vi "Initialize DAQ1.vi"(10 "rate":dbl=1000.0, 11 "number of samples":i32=100) -> (0 "error out":errorcluster, 2 "cDAQ Dev SN":u32, 3 "task out":refnum<k21>)   [LabVIEW 2019]
uses:
  <vilib>/DAQmx/create/channels.llb/DAQmx Create Channel (AI-Voltage-Basic).vi
  <vilib>/DAQmx/create/channels.llb/DAQmx Create Channel (AI-Temperature-Thermocouple).vi
  <vilib>/DAQmx/configure/timing.llb/DAQmx Timing (Sample Clock).vi
  <resource>/objmgr/daqmx.rc
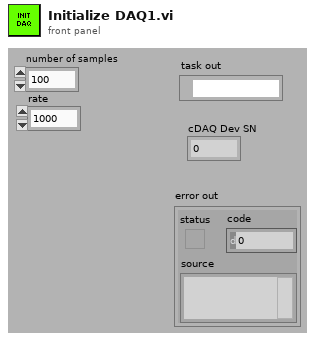
[diagram p1: front panel]
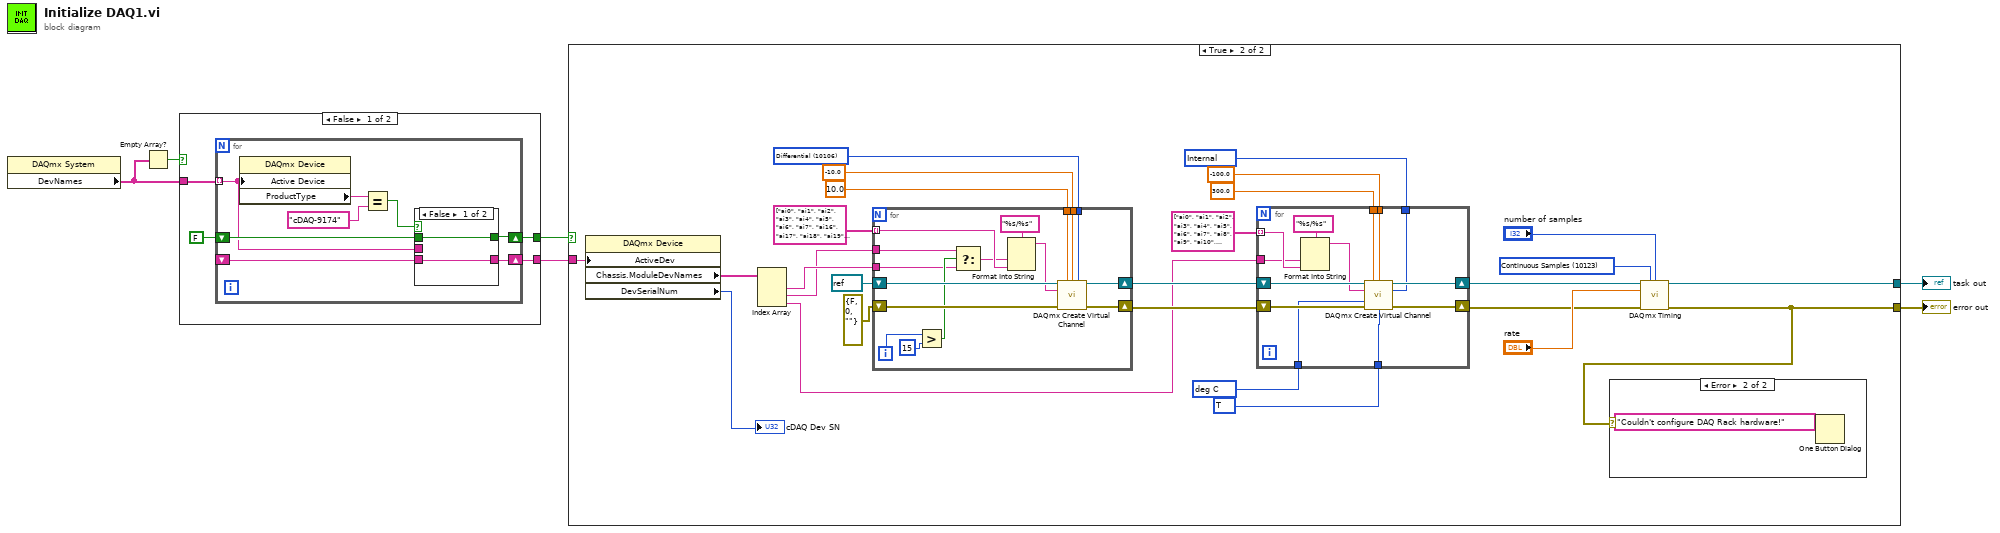
[diagram p0: block diagram]
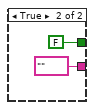
[diagram p3: hidden frame]
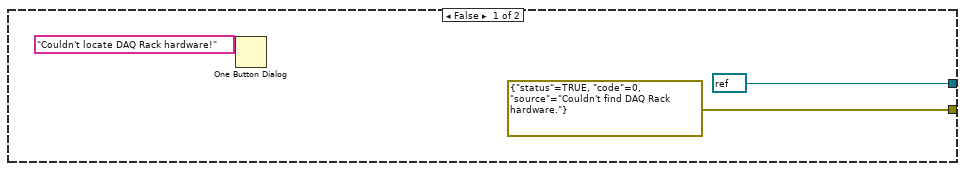
[diagram p4: hidden frame]
diagram:
  n1 = property class="DAQmx System"() -> ("DevNames"=w5:tag[])  [unwired: 2 in, 2 out]
  n2 = Empty Array?(array=w5) -> (empty?=w6:bool)
  n3 = case shown="False" w6 {
    tunnel: w5 -> [w10 _]
    tunnel: [w9 FALSE] -> w4
    tunnel: [w7 tag ""] -> w3
    frame False {
      n4 = for {
        tunnel: w10 -> [w14] mode=indexing
        shift-right: [w16] -> w9
        shift-left: FALSE -> [w15]
        shift-right: [w13] -> w7
        shift-left: _ -> [w12]
        n5 = property class="DAQmx Device"("Active Device"=w14) -> ("ProductType"=w11:string)  [unwired: 2 in, 2 out]
        n6 = Equal?(x=w11, y="cDAQ-9174" ("ProductType")) -> (x = y?=w17:bool)
        n7 = case shown="False" w17 {
          selector: w17 -> [_ w22]
          tunnel: [w20 w22] -> w16
          tunnel: w15 -> [w20 _]
          tunnel: [w19 w21] -> w13
          tunnel: w14 -> [_ w21]
          tunnel: w12 -> [w19 _]
          frame False {
          }
          frame True {
          }
        }
      }
    }
    frame True {
    }
  }
  n8 = case shown="True" w4 {
    tunnel: w3 -> [_ w35]
    tunnel: [refnum<k21> refnum ("task out") w36] -> w2
    tunnel: [errorcluster {"status"=TRUE, "code"=0, "source"="Couldn't find DAQ Rack hardware."} ("error out") w28] -> w1
    frame False {
      n9 = One Button Dialog(message="Couldn't locate DAQ Rack hardware!") -> ()  [unwired: 1 in, 1 out]
    }
    frame True {
      w40 = 10086 items=["J"=10072, "K"=10073, "N"=10077, "R"=10082, "S"=10085, "T"=10086, "B"=10047, "E"=10055] ("thermocouple type")
      w41 = 10143 items=["deg C"=10143, "deg F"=10144, "Kelvins"=10325, "deg R"=10145, "From Custom Scale"=10065] ("units")
      w44 = u32 10200 items=["Internal"=10200, "Constant Value"=10116, "Channel"=10113] ("cjc source")
      w47 = 10106 items=["default"=-1, "RSE"=10083, "NRSE"=10078, "Differential"=10106, "Pseudodifferential"=12529] ("input terminal configuration")
      w50 = 10123 items=["Finite Samples"=10178, "Continuous Samples"=10123, "Hardware Timed Single Point"=12522] ("sample mode")
      n10 = property class="DAQmx Device"("ActiveDev"=w35) -> ("Chassis.ModuleDevNames"=w34:tag[], "DevSerialNum"=→"cDAQ Dev SN":u32)  [unwired: 2 in, 2 out]
      n11 = Index Array(array=w34) -> (element #1=w32:tag, element #2=w31:tag, element #3=w33:tag)  [unwired: 3 in]
      n12 = for {
        tunnel: w47 -> [w82]
        tunnel: -10.0 ("minimum value") -> [w83]
        tunnel: 10.0 ("maximum value") -> [w84]
        tunnel: string[] ["ai0", "ai1", "ai2", "ai3", "ai4", "ai5", "ai6", "ai7", "ai16", "ai17", "ai18", "ai19", "ai20", "ai21", "ai22", "ai23", "ai0", "ai1", "ai2", "ai3", "ai4", "ai5", "ai6", "ai7", "ai16", "ai17", "ai18", "ai19", "ai20", "ai21", "ai22", "ai23"] ("Array") -> [w78] mode=indexing
        shift-right: [w69] -> w54
        shift-left: errorcluster {"status"=FALSE, "code"=0, "source"=""} ("error out") -> [w80]
        shift-right: [w79] -> w53
        shift-left: refnum<k21> refnum ("task out") -> [w81]
        tunnel: w32 -> [w72]
        tunnel: w31 -> [w71]
        i -> [w75]
        n13 = Greater?(x=w75, y=15) -> (0:w73:bool)
        n14 = Select(t=w71, s=w73, f=w72) -> (s? t:f=w70:tag)
        n15 = Format Into String(format string="%s/%s", w70, w78) -> (resulting string=w76:string)  [unwired: 2 in, 1 out]
        n16 = call-poly <vilib>:"DAQmx Create Virtual Channel.vi"("task in"=w81, "maximum value"=w84, "minimum value"=w83, "input terminal configuration"=w82, "physical channels"=w76, "error in"=w80) -> ("task out"=w79:refnum<k21>, "error out"=w69:errorcluster)  [unwired: 8 in]
      }
      n17 = for {
        tunnel: -100.0 ("minimum value") -> [w67]
        tunnel: 300.0 ("maximum value") -> [w68]
        tunnel: w40 -> [w60]
        tunnel: w41 -> [w62]
        tunnel: string[] ["ai0", "ai1", "ai2", "ai3", "ai4", "ai5", "ai6", "ai7", "ai8", "ai9", "ai10", "ai11", "ai12", "ai13", "ai14", "ai15"] ("Array") -> [w58] mode=indexing
        tunnel: w44 -> [w61]
        shift-right: [w63] -> w45
        shift-left: w54 -> [w65]
        shift-right: [w64] -> w46
        shift-left: w53 -> [w66]
        tunnel: w33 -> [w57]
        n18 = Format Into String(format string="%s/%s", w57, w58) -> (resulting string=w56:string)  [unwired: 2 in, 1 out]
        n19 = call-poly <vilib>:"DAQmx Create Virtual Channel.vi"("task in"=w66, "maximum value"=w68, "minimum value"=w67, "physical channels"=w56, "cjc source"=w61, "units"=w62, "error in"=w65, "thermocouple type"=w60) -> ("task out"=w64:refnum<k21>, "error out"=w63:errorcluster)  [unwired: 6 in]
      }
      n20 = call-poly <vilib>:"DAQmx Timing.vi"("task/channels in"=w46, "sample mode"=w50, "samples per channel"="number of samples", "rate"="rate", "error in"=w45) -> ("task out"=w36:refnum<k21>, "error out"=w28:errorcluster)  [unwired: 9 in]
      n21 = case shown="Error" w28 {
        frame No Error {
        }
        frame Error {
          n22 = One Button Dialog(message="Couldn't configure DAQ Rack hardware!") -> ()  [unwired: 1 in, 1 out]
        }
      }
    }
  }
  "task out" <- w2
  "error out" <- w1
